vi "heater current input.vi"(8 "error in (no error)":errorcluster, 9 "heater power":dbl, 10 "heater voltage":dbl, 11 "heater status in":bool) -> (0 "error out":errorcluster, 1 "heater current out":dbl, 3 "heater status out":bool)   [LabVIEW 2014]
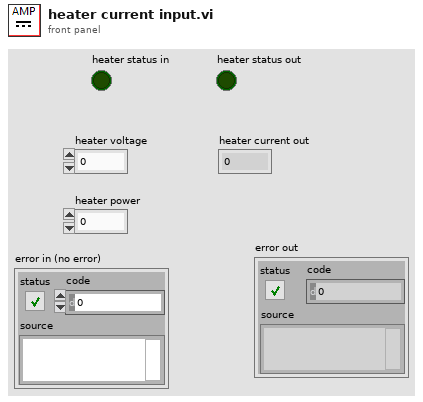
[diagram p1: front panel]
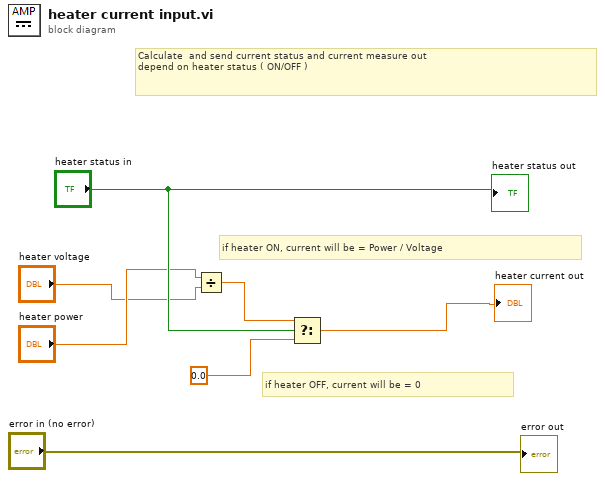
[diagram p0: block diagram]
diagram:
  # "Calculate  and send current status and current measure out\ndepend on heater status ( ON/OFF )"
  # "if heater OFF, current will be = 0"
  # "if heater ON, current will be = Power / Voltage"
  n1 = Divide(x="heater power", y="heater voltage") -> (x/y=w4:dbl)
  n2 = Select(t=w4, s="heater status in", f=0.0) -> (s? t:f=→"heater current out":dbl)
  "heater status out" <- "heater status in"
  "error out" <- "error in (no error)"
